vi "Create.vi"(6 "advanced":T1, 8 "error in (no error)":errorcluster, 11 "queue name":string) -> (0 "error out":errorcluster, 3 "subscriber":refnum<class "IcmMessageSubscriber.lvclass">)   [LabVIEW 2017, in "IcmMessageSubscriber.lvclass"]
doc: "Creates an NI InsightCM Server message bus session."
uses:
  <vilib>/addons/InsightCM/MessageBus/MessageSubscriber/IcmMessageSubscriber.lvclass
  <vilib>/addons/InsightCM/MessageBus/MessageSubscriber/controls/SubscriberAdvancedConfig.ctl
  <vilib>/addons/InsightCM/MessageBus/MessageSubscriber/controls/MessageSubscriberData.ctl
  C:/Program Files (x86)/National Instruments/LabVIEW 2017/vi.lib/addons/InsightCM/Binaries/LabviewMessageAdapter.dll
  Binaries/LabviewMessageAdapter.dll
  <vilib>/addons/InsightCM/MessageBus/MessageSubscriber/IcmMessageSubscriber.lvclass/IcmMessageSubscriber.ctl
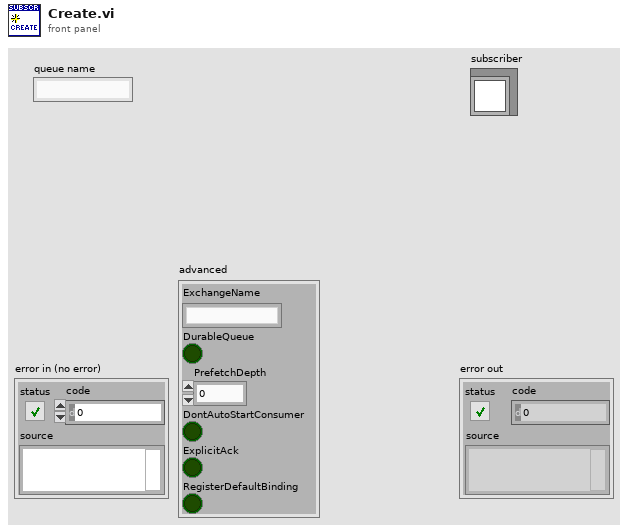
[diagram p1: front panel]
types:
  T1 = typedef "SubscriberAdvancedConfig.ctl" = cluster{"ExchangeName":string, "DurableQueue":bool, "PrefetchDepth":u16, "DontAutoStartConsumer":bool, "ExplicitAck":bool, "RegisterDefaultBinding":bool}
  T2 = typedef "MessageSubscriberData.ctl" = cluster{"Subscriber":refnum<k24>}
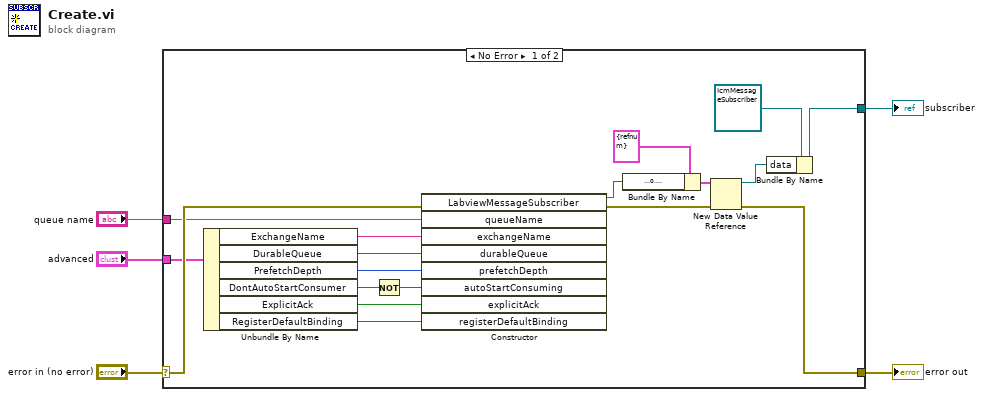
[diagram p0: block diagram]
diagram:
  n1 = case shown="No Error" "error in (no error)" {
    selector: "error in (no error)" -> [w19 w24]
    tunnel: [w18 w24] -> w4
    tunnel: [w20 _] -> w3
    tunnel: "advanced" -> [w16 _]
    tunnel: "queue name" -> [w10 _]
    frame No Error {
      n2 = Unbundle By Name(w16) -> ("ExchangeName"=w12:string, "DurableQueue"=w13:bool, "PrefetchDepth"=w14:u16, "DontAutoStartConsumer"=w15:bool, "ExplicitAck"=w7:bool, "RegisterDefaultBinding"=w6:bool)
      n3 = Not(x=w15) -> (.not. x?=w11:bool)
      n4 = constructor class="LabviewMessageSubscriber"(error in=w19, "queueName"=w10, "exchangeName"=w12, "durableQueue"=w13, "prefetchDepth"=w14, "autoStartConsuming"=w11, "explicitAck"=w7, "registerDefaultBinding"=w6) -> (reference out=w9:refnum<k24>, error out=w22:errorcluster)  [unwired: 2 in, 8 out]
      n5 = Bundle By Name(cluster=T2 {"Subscriber"=refnum} ("Subscriber"), "Subscriber"=w9) -> (w23:T2)
      n6 = New Data Value Reference(data value=w23, error in=w22) -> (data value reference=w8:refnum<data-value>, error out=w18:errorcluster)
      n7 = Bundle By Name(cluster=refnum<class "IcmMessageSubscriber.lvclass"> refnum ("IcmMessageSubscriber out"), "data"=w8) -> (w20:refnum<class "IcmMessageSubscriber.lvclass">)
    }
    frame Error {
    }
  }
  "error out" <- w4
  "subscriber" <- w3
